vi "Get PID Gains from Schedule.vi"(10 "Parameter Refs":refnum<data-value>[](array[refnum]), 11 "Gain Schedule Value":dbl[](array[numeric])) -> (2 "Parameter Refs":refnum<data-value>[](array[refnum]), 3 "PID":T1(array[cluster]))   [LabVIEW 2019, in "Control Addon Engine.lvlib"]
uses:
  Control Addon Engine.lvlib
  Shared/Types/Gain Schedule.ctl
  <vilib>/addons/control/pid/pid.llb/PID Gain Schedule (DBL).vi
  <vilib>/addons/control/pid/NI_PID_pid.lvlib
  Shared/Control Addon Shared.lvlib
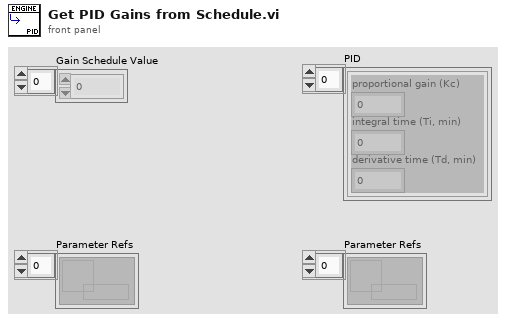
[diagram p1: front panel]
types:
  T1 = cluster{"proportional gain (Kc)":dbl, "integral time (Ti, min)":dbl, "derivative time (Td, min)":dbl}[]
  T2 = typedef "Simple PID Addon Shared.lvlib/Gain Schedule.ctl" = cluster{"Gain Schedule":cluster{"PID gains":cluster{"proportional gain (Kc)":dbl, "integral time (Ti, min)":dbl, "derivative time (Td, min)":dbl}, "max value":dbl}[]}
  T3 = cluster{"PID gains":cluster{"proportional gain (Kc)":dbl, "integral time (Ti, min)":dbl, "derivative time (Td, min)":dbl}, "max value":dbl}[]
  T4 = cluster{"proportional gain (Kc)":dbl, "integral time (Ti, min)":dbl, "derivative time (Td, min)":dbl}
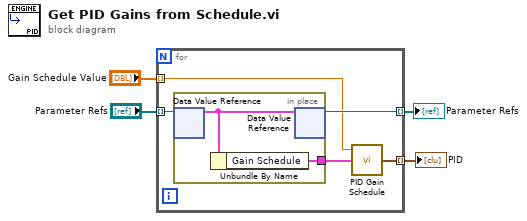
[diagram p0: block diagram]
diagram:
  n1 = for {
    tunnel: [w9] -> w3 mode=indexing
    tunnel: "Parameter Refs" -> [w8] mode=indexing
    tunnel: [w6] -> w1 mode=indexing
    tunnel: "Gain Schedule Value" -> [w5] mode=indexing
    n2 = in-place {
      in-place-border: [w10] -> w7
      n3 = in-place-dvr #1(w8) -> (w11:T2)  [unwired: 1 out]
      n4 = Unbundle By Name(w11) -> ("Gain Schedule"=w10:T3)
      n5 = in-place-dvr #1(w11) -> (w6:refnum<data-value>)  [unwired: 1 out]
    }
    n6 = call-poly <vilib>:"PID Gain Schedule.vi"("PID gain schedule"=w7, "gain scheduling value"=w5) -> ("PID gains out"=w9:T4)  [unwired: 2 in, 1 out]
  }
  "PID" <- w3
  "Parameter Refs" <- w1
